vi "FPGA_PPG_query_revision.vi"(0 "resource_in":refnum<visa-resource-name>, 5 "error in (no error)":errorcluster) -> (14 "resource_out":refnum<visa-resource-name>, 16 "revision":string, 19 "error out":errorcluster)   [LabVIEW 2014, in "NI-FPGA_PPG_Driver.lvlib"]
doc: "Queries the revision number (firmware revision) of the FPGA code.\n\nDietrich Beck, GSI Helmholtzzentrum fuer Schwerionenforschung, Germany"
uses:
  NI-FPGA_PPG_Driver.lvlib
  FPGA_PPG_action_type.ctl
  <vilib>/Utility/error.llb/Error Cluster From Error Code.vi
  <vilib>/rvi/errors/niLvFpgaAdjustHostInterfaceError.vi
  <vilib>/rvi/interface/nirviReadWriteControl/nirviReadWriteControl.xnode
  FPGA_PPG_vi_ref.ctl
  FPGA Bitfiles/NI-FPGA-PPG.lvproj_PCI-7811R_FPGA_target_main.vi.lvbitx
  NiFpgaLv.dll
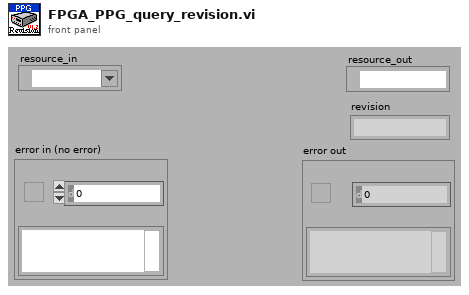
[diagram p1: front panel]
types:
  T1 = typedef "NI-FPGA_PPG_Driver.lvlib/FPGA_PPG_action_type.ctl" = enum16{"GET", "SET", "REMOVE"}
  T2 = typedef "NI-FPGA_PPG_Driver.lvlib/FPGA_PPG_vi_ref.ctl" = refnum<k20>
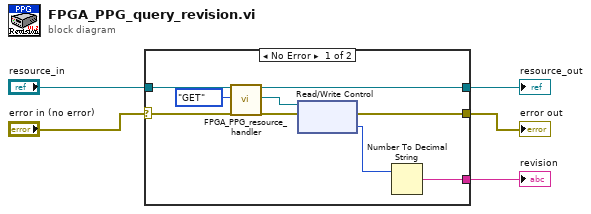
[diagram p0: block diagram]
diagram:
  n1 = case shown="No Error" "error in (no error)" {
    selector: "error in (no error)" -> [w13 w16]
    tunnel: [w10 w16] -> w4
    tunnel: "resource_in" -> [w14 w15]
    tunnel: [w11 w15] -> w2
    tunnel: [w9 _] -> w1
    frame No Error {
      n2 = call "FPGA_PPG_resource_handler.vi"("resource_in"=w14, "action"=FPGA_PPG_action_type."GET", "error in (no error)"=w13) -> ("resource_out"=w11:refnum<visa-resource-name>, "FPGA VI Reference Out"=w7:T2, "error out"=w12:errorcluster)  [unwired: 14 in]
      n3 = xnode "Read/Write Control"("FPGA VI Reference In"=w7, "error in"=w12) -> ("error out"=w10:errorcluster, "revision"=w8:i32)  [unwired: 1 out]
      n4 = Number To Decimal String(number=w8) -> (decimal integer string=w9:string)  [unwired: 1 in]
    }
    frame Error {
    }
  }
  "error out" <- w4
  "resource_out" <- w2
  "revision" <- w1
